vi "zlgcan_demo_EU.vi"() -> ()   [LabVIEW 2018]
doc: "演示例子，适用的设备：PCI-5010-U、PCI-5020-U、USBCAN-E-U、USBCAN-2E-U、USBCAN-4E-U、USBCAN-8E-U、CANalyst-II+"
uses:
  data_type/ZCAN_InitCAN_setting_EU.ctl
panel:
  in  "工作模式":u8(ring) items=["正常", "只听"]
  in  "自定义波特率字符输入":string
  in  "使用自定义波特率？":bool
  in  "波特率":u32(ring)=500000 items=["1Mbps"=1000000, "800kbps"=800000, "500kbps"=500000, "250kbps"=250000, "125kbps"=125000, "100kbps"=100000, "50kbps"=50000]
  in  "通道索引":u32(ring) items=["0", "1", "2", "3"]
  in  "设备索引":u32(ring) items=["0", "1", "2", "3"]
  in  "设备类型":u32(ring)=21 items=["PCI-9810"=2, "USBCAN-II"=4, "PCI-5010-U"=19, "USBCAN-E-U"=20, "USBCAN-2E-U"=21, "PCI-5020-U"=22, "USBCAN-4E-U"=31, "USBCAN-8E-U"=34, "USBCANFD-100U"=42, "USBCANFD-200U"=41, "PCIE-CANFD-100U"=38, "PCIE-CANFD-200U"=39, "PCIE-CANFD-400U"=40, "云设备"=46]
  in  "开启CAN":bool
  in  "stop":bool
  in  "ID":u32 format="0x%08x"
  in  "数据长度(最大8字节)":u8=8 max=8
  in  "Data Byte 8":u8 caption="data88" format="%.0x"
  in  "Data Byte 7":u8 caption="data7" format="%.0x"
  in  "Data Byte 6":u8 caption="data6" format="%.0x"
  in  "Data Byte 5":u8 caption="data5" format="%.0x"
  in  "Data Byte 4":u8 caption="data4" format="%.0x"
  in  "Data Byte 3":u8 caption="data3" format="%.0x"
  in  "Data Byte 2":u8 caption="data2" format="%.0x"
  in  "Data Byte 1":u8 caption="data1" format="%.0x"
  in  "帧格式":u32(ring) items=["数据帧", "远程帧"]
  in  "发送方式":u32(ring) items=["正常发送", "单次发送", "自发自收", "单次自发自收"]
  in  "帧类型":u32(ring) items=["标准帧", "扩展帧"]
  in  "每次发送帧数":u32=1
  in  "发送":bool
  in  "ZCAN_InitCAN_Setting_EU":T1
  out "can_index_handle(out)":u32
  out "Device_handle(out)":u32
  out "已接收帧数":u32
  out "接收字符串显示":string caption="String"
  # "停止程序前，需要先关闭CAN卡"
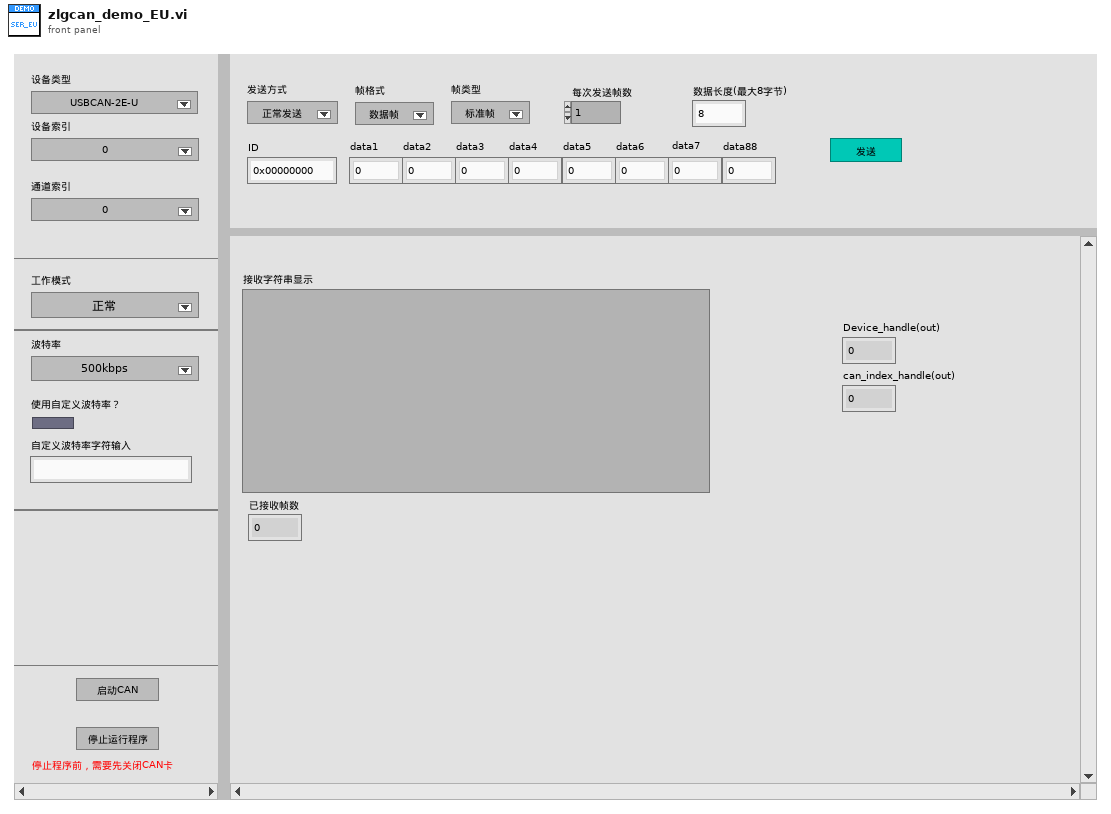
[diagram p1: front panel]
types:
  T1 = typedef "ZCAN_InitCAN_setting_EU.ctl" = cluster{"baudrate":u32, "baud_rate_custom？":bool, "RateCustom":string, "mode":u8}
  T2 = cluster{"[0]":u8, "[1]":u8, "[2]":u8, "[3]":u8, "[4]":u8, "[5]":u8, "[6]":u8, "[7]":u8}
  T3 = cluster{u32, u8, u8, u8, u8, cluster{"[0]":u8, "[1]":u8, "[2]":u8, "[3]":u8, "[4]":u8, "[5]":u8, "[6]":u8, "[7]":u8}, u64}[]
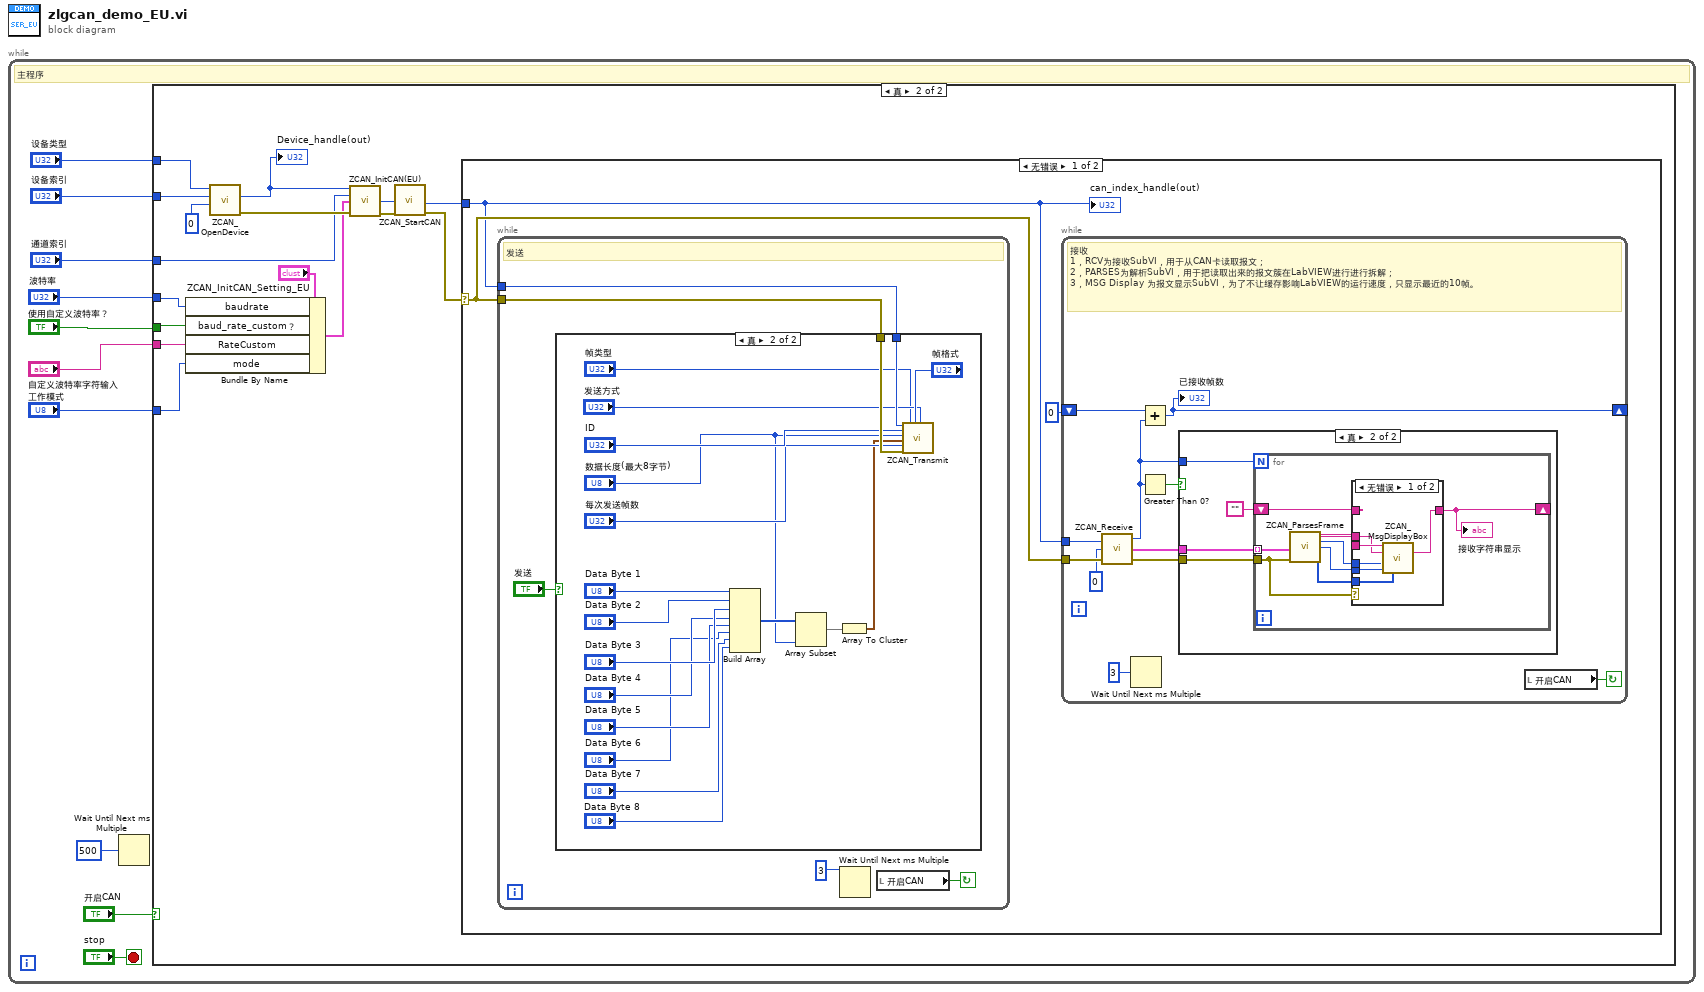
[diagram p0: block diagram]
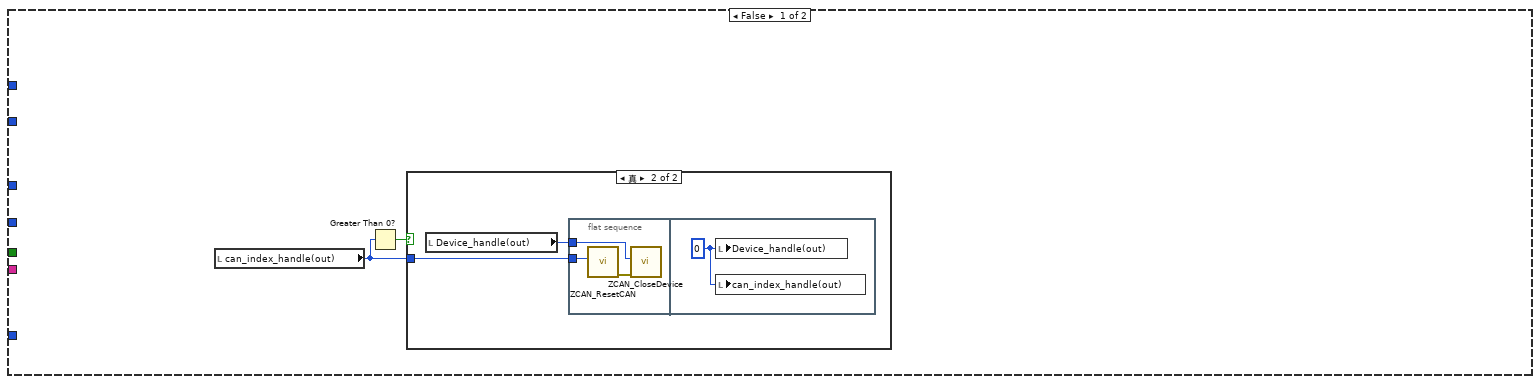
[diagram p2: hidden frame]
diagram:
  n1 = while {
    stop <- "stop" stop-if-true
    # "主程序"
    n2 = Wait Until Next ms Multiple(millisecond multiple=u32 500) -> ()  [unwired: 1 out]
    n3 = case shown="真" "开启CAN" {
      tunnel: "通道索引" -> [_ w25]
      tunnel: "波特率" -> [_ w22]
      tunnel: "使用自定义波特率？" -> [_ w21]
      tunnel: "自定义波特率字符输入" -> [_ w20]
      tunnel: "工作模式" -> [_ w19]
      tunnel: "设备类型" -> [_ w30]
      tunnel: "设备索引" -> [_ w31]
      frame False {
        # "关闭CAN卡"
        n4 = local read "can_index_handle(out)"() -> (w11:u32)
        n5 = Greater Than 0?(x=w11) -> (x > 0?=w12:bool)
        n6 = case shown="真" w12 {
          tunnel: w11 -> [_ w14]
          frame False {
          }
          frame True {
            n7 = local read "Device_handle(out)"() -> (w13:u32)
            n8 = flat-sequence {
              tunnel: w14 -> [w16]
              tunnel: w13 -> [w15]
              frame #0 {
                n9 = call "ZCAN_ResetCAN.vi"("can_handle"=w16) -> ("error out"=w17:errorcluster)  [unwired: 9 in, 1 out]
                n10 = call "ZCAN_CloseDevice.vi"("error in (no error)"=w17, "device_handle"=w15) -> ()  [unwired: 8 in, 2 out]
              }
              frame #1 {
                w18 = u32 0 ("can_index_handle(out)")
                n11 = local write "Device_handle(out)"(w18) -> ()
                n12 = local write "can_index_handle(out)"(w18) -> ()
              }
            }
          }
        }
      }
      frame True {
        n13 = Bundle By Name(cluster="ZCAN_InitCAN_Setting_EU", "baudrate"=w22, "baud_rate_custom？"=w21, "RateCustom"=w20, "mode"=w19) -> (w23:T1)
        n14 = call "ZCAN_OpenDevice.vi"("reserved"=0, "device_index"=w31, "device_type"=w30) -> ("error out"=w29:errorcluster, "DEVICE_HANDLE"=w26:u32)  [unwired: 7 in]
        "Device_handle(out)" <- w26
        n15 = call "ZCAN_InitCAN(EU).vi"("device_hande"=w26, "can_index"=w25, "ZCAN_InitCAN_Setting_EU"=w23, "error in (no error)"=w29) -> ("can_index_handle"=w32:u32, "error out"=w33:errorcluster)  [unwired: 10 in]
        n16 = call "ZCAN_StartCAN.vi"("error in (no error)"=w33, "can_index_handle"=w32) -> ("error out"=w27:errorcluster, "can_index_handle(out)"=w28:u32)  [unwired: 7 in, 1 out]
        n17 = case shown="无错误" w27 {
          selector: w27 -> [w36 _]
          tunnel: w28 -> [w35 _]
          frame No Error {
            n18 = while {
              tunnel: w35 -> [w71]
              tunnel: w36 -> [w69]
              stop <- w70 continue-if-true
              # "发送"
              n19 = case shown="真" "发送" {
                tunnel: w71 -> [_ w92]
                tunnel: w69 -> [_ w91]
                frame False {
                }
                frame True {
                  n20 = Build Array("Data Byte 1", "Data Byte 2", "Data Byte 3", "Data Byte 4", "Data Byte 5", "Data Byte 6", "Data Byte 7", "Data Byte 8") -> (w78:u8[])
                  n21 = Array Subset(array=w78, length="数据长度(最大8字节)") -> (w76:u8[])  [unwired: 1 in]
                  n22 = Array To Cluster(array=w76) -> (cluster=w75:T2)
                  n23 = call "ZCAN_Transmit.vi"("can_index_handle"=w92, "ID"="ID", "数据长度"="数据长度(最大8字节)", "DATA"=w75, "每次发送帧数"="每次发送帧数", "error in (no error)"=w91, "帧类型"="帧类型", "帧格式"="帧格式", "发送方式"="发送方式") -> ()  [unwired: 10 in, 1 out]
                }
              }
              n24 = Wait Until Next ms Multiple(millisecond multiple=u32 3) -> ()  [unwired: 1 out]
              n25 = local read "开启CAN"() -> (w70:bool)
            }
            n26 = while {
              tunnel: w36 -> [w45]
              tunnel: w35 -> [w43]
              shift-right: [w46] -> _
              shift-left: 0 -> [w47]
              stop <- w38 continue-if-true
              # "接收\n1，RCV为接收SubVI，用于从CAN卡读取报文；\n2，PARSES为解析SubVI，用于把读取出来的报文簇在LabVIEW进行进行拆解；\n3，MSG Display 为报文显示SubVI，为了不让缓存影响LabVIEW的运行速度，只显示最近的10帧。"
              n27 = call "ZCAN_Receive.vi"("error in (no error)"=w45, "type"=u8 0, "can_handle"=w43) -> ("error out"=w41:errorcluster, "Receive"=w42:T3, "Receive_Num"=w40:u32)
              n28 = Wait Until Next ms Multiple(millisecond multiple=u32 3) -> ()  [unwired: 1 out]
              n29 = Add(x=w47, y=w40) -> (x+y=w46:u32)
              "已接收帧数" <- w46
              n30 = Greater Than 0?(x=w40) -> (x > 0?=w39:bool)
              n31 = case shown="真" w39 {
                tunnel: w40 -> [_ w52]
                tunnel: w42 -> [_ w51]
                tunnel: w41 -> [_ w50]
                frame False {
                }
                frame True {
                  n32 = for {
                    N: w52 -> [_]
                    tunnel: w51 -> [w59] mode=indexing
                    tunnel: w50 -> [w58]
                    shift-right: [w61] -> _
                    shift-left: "" -> [w60]
                    n33 = call "ZCAN_ParsesFrame.vi"("ZCAN_Receive_Data"=w59, "error in (no error)"=w58) -> ("帧格式"=w53:string, "帧类型"=w54:string, "ID"=w55:u32, "data_len"=w57:u8, "data"=w56:u8[])  [unwired: 8 in, 1 out]
                    n34 = case shown="无错误" w58 {
                      tunnel: [w67 w68] -> w61
                      tunnel: w60 -> [_ w68]
                      tunnel: w57 -> [w66 _]
                      tunnel: w56 -> [w65 _]
                      tunnel: w55 -> [w64 _]
                      tunnel: w54 -> [w63 _]
                      tunnel: w53 -> [w62 _]
                      frame No Error {
                        n35 = call "ZCAN_MsgDisplayBox.vi"("帧类型"=w63, "ID"=w64, "帧格式"=w62, "Message Data"=w65, "data_len"=w66) -> ("Output String"=w67:string)  [unwired: 10 in]
                      }
                      frame Error {
                      }
                    }
                    "接收字符串显示" <- w61
                  }
                }
              }
              n36 = local read "开启CAN"() -> (w38:bool)
            }
            "can_index_handle(out)" <- w35
          }
          frame Error {
          }
        }
      }
    }
  }
